vi "LowShooter Controller.vi"(8 "error in":errorcluster) -> ()   [LabVIEW 2015]
doc: "This VI executes continuously carrying out the current operation and responding to updates or new operations. It will often contain the timing or control code that is difficult to place directly in TeleOp. This VI generally opens all sensors and motors and isolates the rest of the robot code from knowing how the operations are carried out."
uses:
  LowShooter Operations.ctl
  <vilib>/Rock Robotics/WPI/CAN/TalonSRX/WPI_CANTalonSRX_GlobalStatus.ctl
  LowShooter Setpoints.ctl
  Framework/Motor Ref Names Type Def.ctl
  Solenoids/Solenoids.ctl
  <vilib>/Rock Robotics/WPI/Solenoid/WPI_SolenoidValue.ctl
  Framework/Robot Global Data.vi
  Shooter Global.vi
panel:
  out "Talon SRX Status":T1
  in  "OK Button":bool
  in  "Ball Seen":dbl
  out "Arm Down":bool
  out "Operation":T2
  out "Back Switch":bool
  out "Ball Present":bool
  out "error out":errorcluster
  in  "error in":errorcluster
  out "Current\nCmd 2":string
  out "Current\nCmd":string
  # "Tip: It may be helpful to observe inputs and sensor values.\nYou may also want to display tuning or debugging controls."
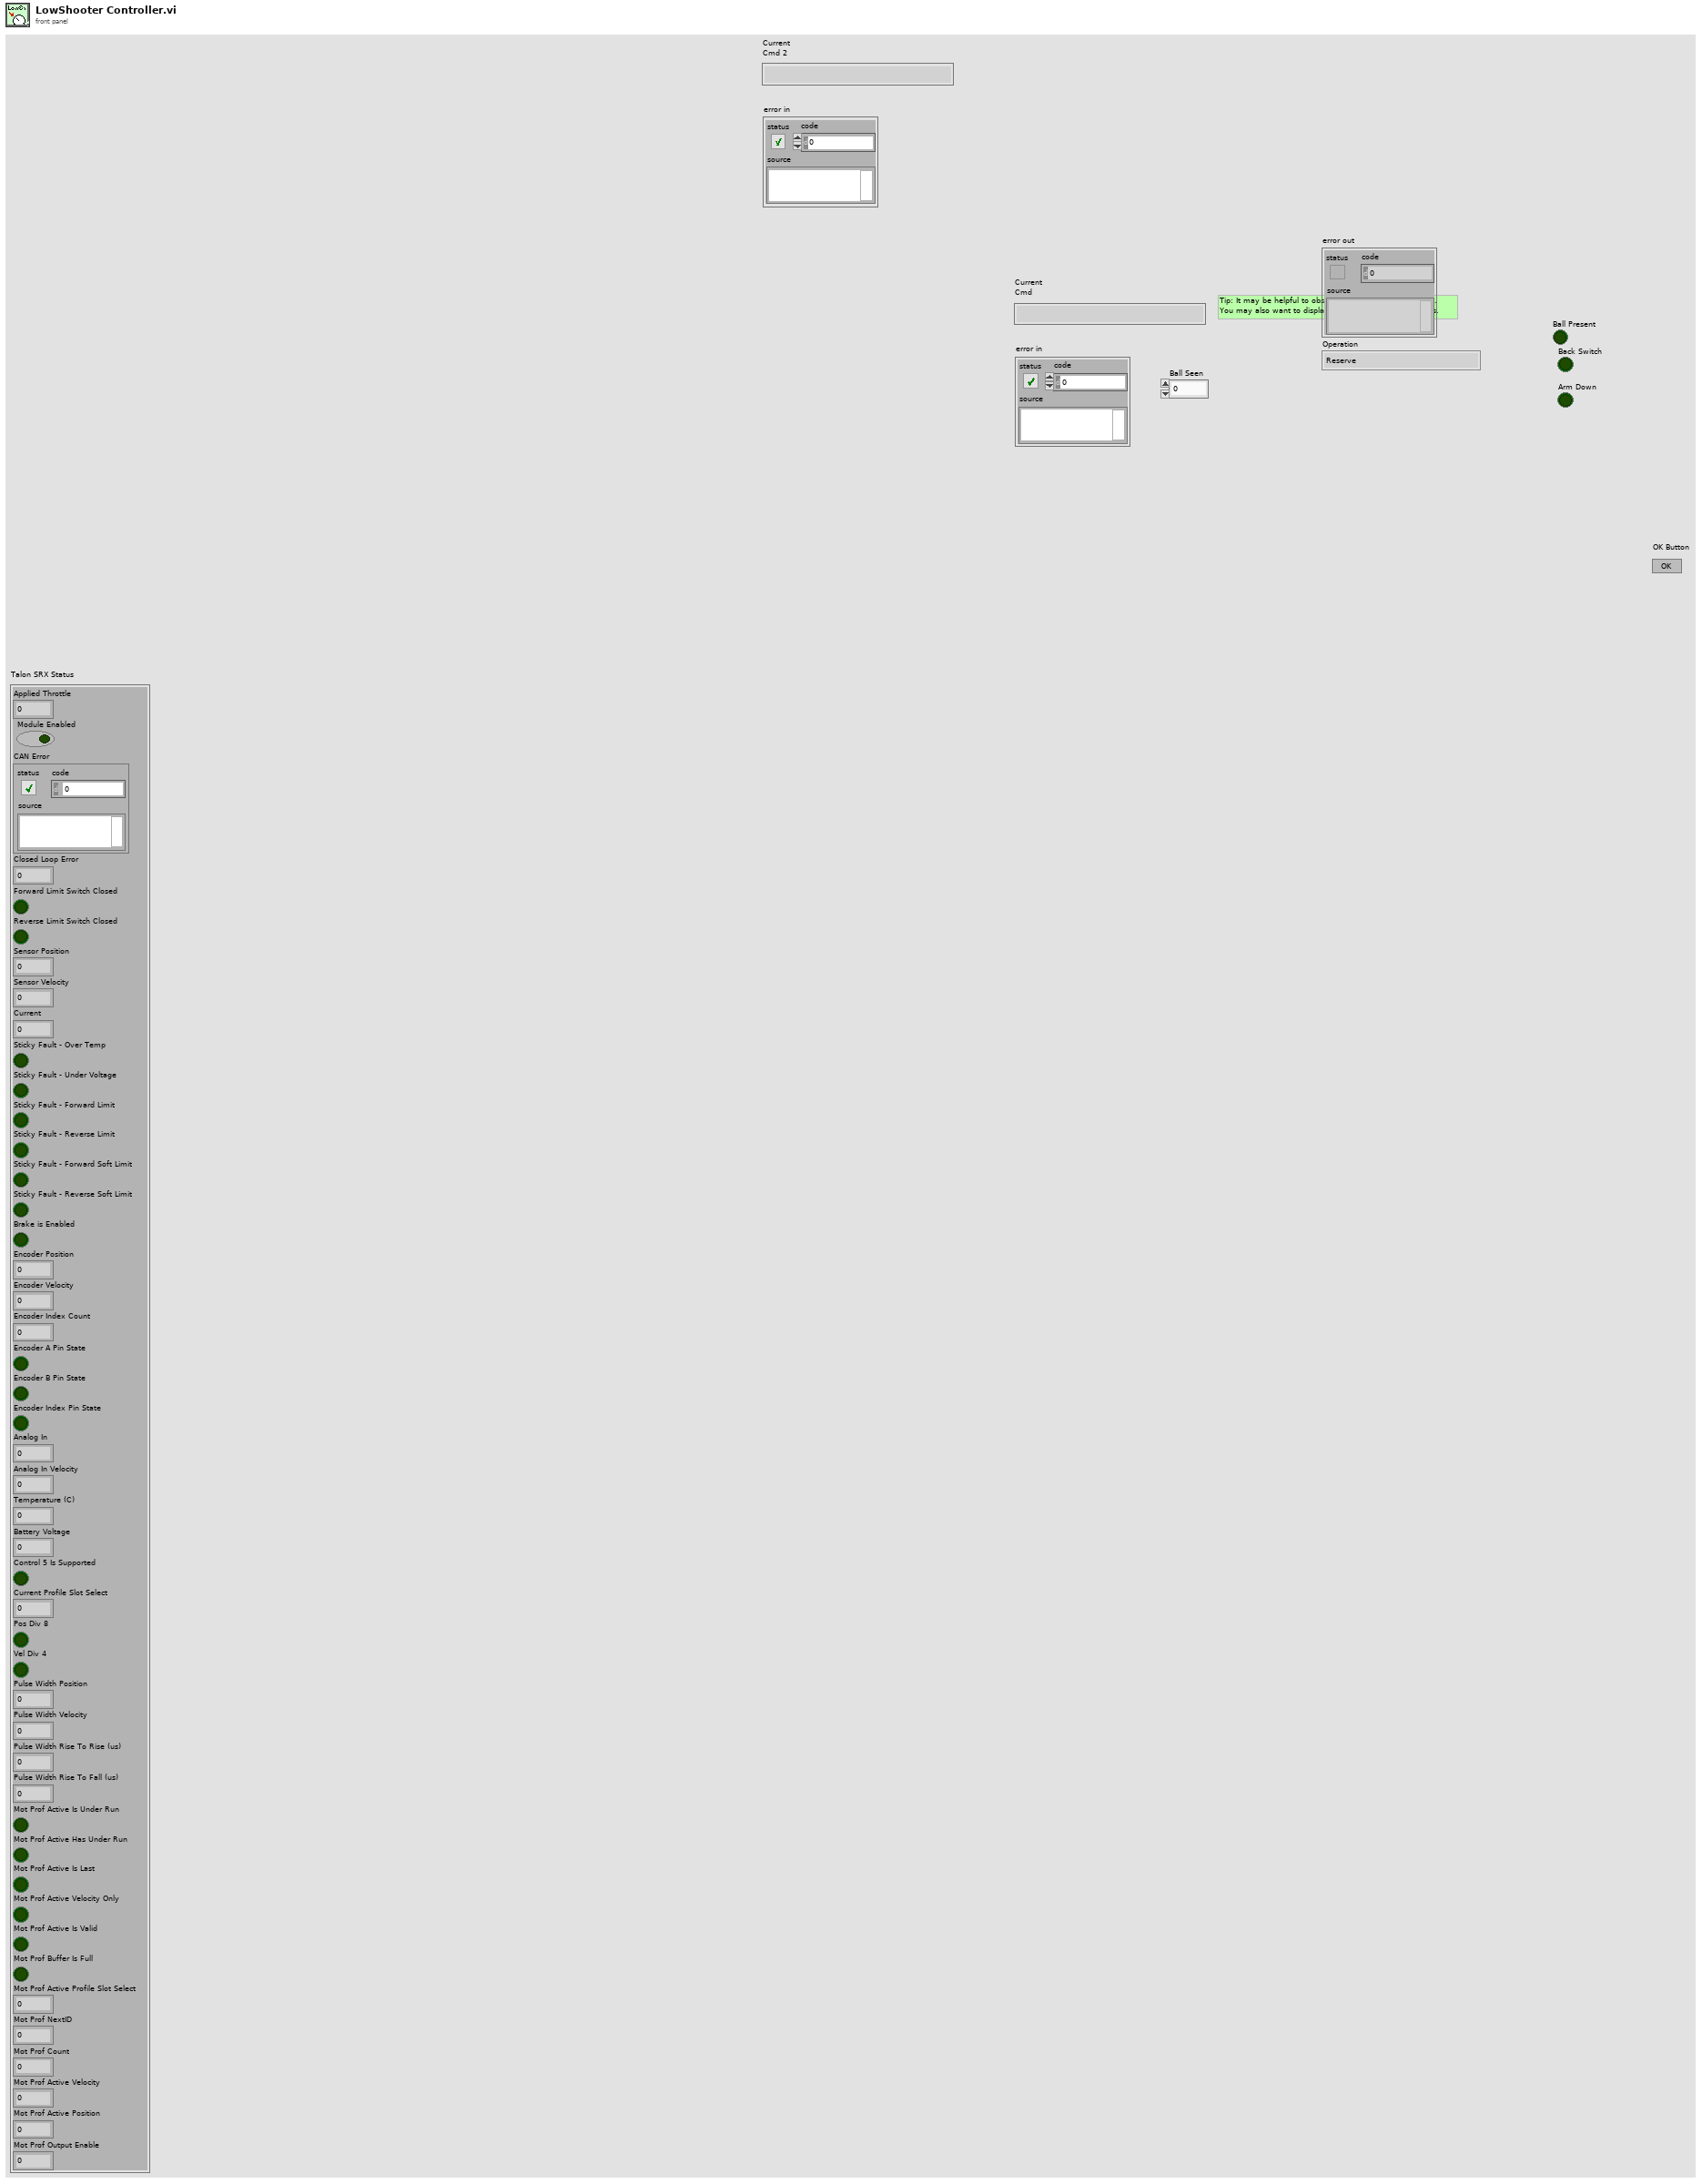
[diagram p1: front panel]
types:
  T1 = typedef "WPI_CANTalonSRX_GlobalStatus.ctl" = cluster{"Applied Throttle":dbl, "Module Enabled":bool, "CAN Error":errorcluster, "Closed Loop Error":dbl, "Forward Limit Switch Closed":bool, "Reverse Limit Switch Closed":bool, "Sensor Position":dbl, "Sensor Velocity":dbl, "Current":dbl, "Sticky Fault - Over Temp":bool, "Sticky Fault - Under Voltage":bool, "Sticky Fault - Forward Limit":bool, "Sticky Fault - Reverse Limit":bool, "Sticky Fault - Forward Soft Limit":bool, "Sticky Fault - Reverse Soft Limit":bool, "Brake is Enabled":bool, "Encoder Position":dbl, "Encoder Velocity":dbl, "Encoder Index Count":dbl, "Encoder A Pin State":bool, "Encoder B Pin State":bool, "Encoder Index Pin State":bool, "Analog In":dbl, "Analog In Velocity":dbl, "Temperature (C)":dbl, "Battery Voltage":dbl, "Control 5 Is Supported":bool, "Current Profile Slot Select":dbl, "Pos Div 8":bool, "Vel Div 4":bool, "Pulse Width Position":i32, "Pulse Width Velocity":i32, "Pulse Width Rise To Rise (us)":i32, "Pulse Width Rise To Fall (us)":i32, "Mot Prof Active Is Under Run":bool, "Mot Prof Active Has Under Run":bool, "Mot Prof Active Is Last":bool, "Mot Prof Active Velocity Only":bool, "Mot Prof Active Is Valid":bool, "Mot Prof Buffer Is Full":bool, "Mot Prof Active Profile Slot Select":i32, "Mot Prof NextID":i32, "Mot Prof Count":i32, "Mot Prof Active Velocity":dbl, "Mot Prof Active Position":dbl, "Mot Prof Output Enable":i32}
  T2 = typedef "LowShooter Operations.ctl" = enum16{"Reserve", "Read Current", "Immediate", "Shoot", "Retrieve", "Move Arm Down", "Move Arm"}
  T3 = typedef "Robot Type Def.ctl" = enum32{"Disabled", "Ghost", "Casper", "Lofty", "Board", "RaceRobot"}
  T4 = typedef "Motor Ref Names Type Def.ctl" = enum16{"Angular Motor", "Shooter Motor Bottom", "Shooter Motor Top", "Arm Shooter Motor"}
  T5 = typedef "WPI_SolenoidValue.ctl" = enum16{"Off", "On", "Forward", "Reverse"}
  T6 = typedef "Solenoids.ctl" = enum16{"Gear Low", "Gear High", "Shoot Ball", "Hold Ball", "PTO Active", "PTO De-Active"}
  T7 = typedef "LowShooter Setpoints.ctl" = cluster{"Operation":T2, "Setpoint":dbl, "Duration":dbl}
  T8 = typedef "Motor Ref Array Type Def.ctl" = T9[]
  T9 = typedef "Detailed Motor Type Def.ctl" = cluster{"MotorRef":T10, "Encoder Ticks Per Rev":dbl, "Set Position":dbl}
  T10 = typedef "WPI_MotorControlDeviceRef.ctl" = cluster{"DeviceStatus":errorcluster, "Type":T11, "PWM":cluster{"PWM Channel":T12, "DeadBand":T13}, "CAN":cluster{"Device Number":u8, "Control Mode":T14, "Semaphore":T15, "Max Vout":dbl, "TalonSRX Control Mode":T16}, "Invert":bool}
  T11 = typedef "WPI_MotorControlType.ctl" = enum16{"PWM", "CAN", "CANTalonSRX"}
  T12 = typedef "FPGA_DIOPWMChannel.ctl" = enum8{"PWM 0", "PWM 1", "PWM 2", "PWM 3", "PWM 4", "PWM 5", "PWM 6", "PWM 7", "PWM 8", "PWM 9", "PWM MXP 0", "PWM MXP 1", "PWM MXP 2", "PWM MXP 3", "PWM MXP 4", "PWM MXP 5", "PWM MXP 6", "PWM MXP 7", "PWM MXP 8", "PWM MXP 9", "Invalid"}
  T13 = typedef "WPI_PWMDeadband.ctl" = cluster{"Name":string, "maxPositivePwm":i32, "minPositivePwm":i32, "centerPwm":i32, "maxNegativePwm":i32, "minNegativePwm":i32, "angularRange":u16}
  T14 = typedef "WPI_CANJaguar_ControlMode.ctl" = enum8{"Percent VBus", "Current", "Speed", "Position", "Voltage"}
  T15 = typedef "Semaphore RefNum" = refnum<k1>
  T16 = typedef "WPI_CANTalonSRX_APIControlMode.ctl" = enum8{"Percent VBus", "Speed", "Position", "Slave", "Unchanged / Invalid", "Voltage Compensation", "Current", "Motion Profile"}
  T17 = typedef "Command Status Info.ctl" = cluster{"Name":string, "Status":T18, "notifier out":T19}
  T18 = typedef "Completion Status.ctl" = enum16{"Successful", "Aborted", "Incomplete"}
  T19 = typedef "Completion Notifier.ctl" = refnum<notifier>
  T20 = cluster{"Default Command":T7, "Command Timing":cluster{"Start Time (ms)":u32, "Iterations":i32}, "Command Arguments":cluster{"Command Info":T17, "Description":string, "Default Command":T7, "notifier out":refnum<notifier>, "Subsystem Name":string}}
  T21 = typedef "Addon Motor Type Def.ctl" = cluster{"SwitchDevRef":T22, "LidarRef":T25, "Arm Sensors":cluster{"Front Sensor":T22, "Back Sensor":T22, "Ball Sensor":T22}}
  T22 = typedef "WPI_SwitchDevRef.ctl" = cluster{"DevStatus":errorcluster, "DIO Channel":T23, "CntIndex":T24, "Normally Closed":bool}
  T23 = typedef "FPGA_DIOChannel.ctl" = enum8{"DIO 0", "DIO 1", "DIO 2", "DIO 3", "DIO 4", "DIO 5", "DIO 6", "DIO 7", "DIO 8", "DIO 9", "DIO MXP 0", "DIO MXP 1", "DIO MXP 2", "DIO MXP 3", "DIO MXP 4", "DIO MXP 5", "DIO MXP 6", "DIO MXP 7", "DIO MXP 8", "DIO MXP 9", "DIO MXP 10", "DIO MXP 11", "DIO MXP 12", "DIO MXP 13", "DIO MXP 14", "DIO MXP 15", "Invalid"}
  T24 = typedef "FPGA_CounterCtrSystemIndex.ctl" = enum8{"Ctr 0", "Ctr 1", "Ctr 2", "Ctr 3", "Ctr 4", "Ctr 5", "Ctr 6", "Ctr 7", "Invalid"}
  T25 = typedef "Lidar Type Def.ctl" = cluster{"I2CDevRef":T26}
  T26 = typedef "WPI_I2CDevRef.ctl" = cluster{"DevStatus":errorcluster, "Device Address":u8, "Handle":i32, "I2C Bus":T27}
  T27 = typedef "i2c_bus.ctl" = enum16{"I2C On-Board", "I2C MXP", "Invalid"}
  T28 = typedef "Shooter Settings Type Def.ctl" = cluster{"Bottom Roller Out Speed":dbl, "Top Roller Out Speed":dbl, "Bottom Roller In Speed":dbl, "Top Roller In Speed":dbl, "Intake Time Limit":dbl, "Intake Close Claw Delay":dbl, "Shoot Delay":dbl, "Shoot Follow Through":dbl}
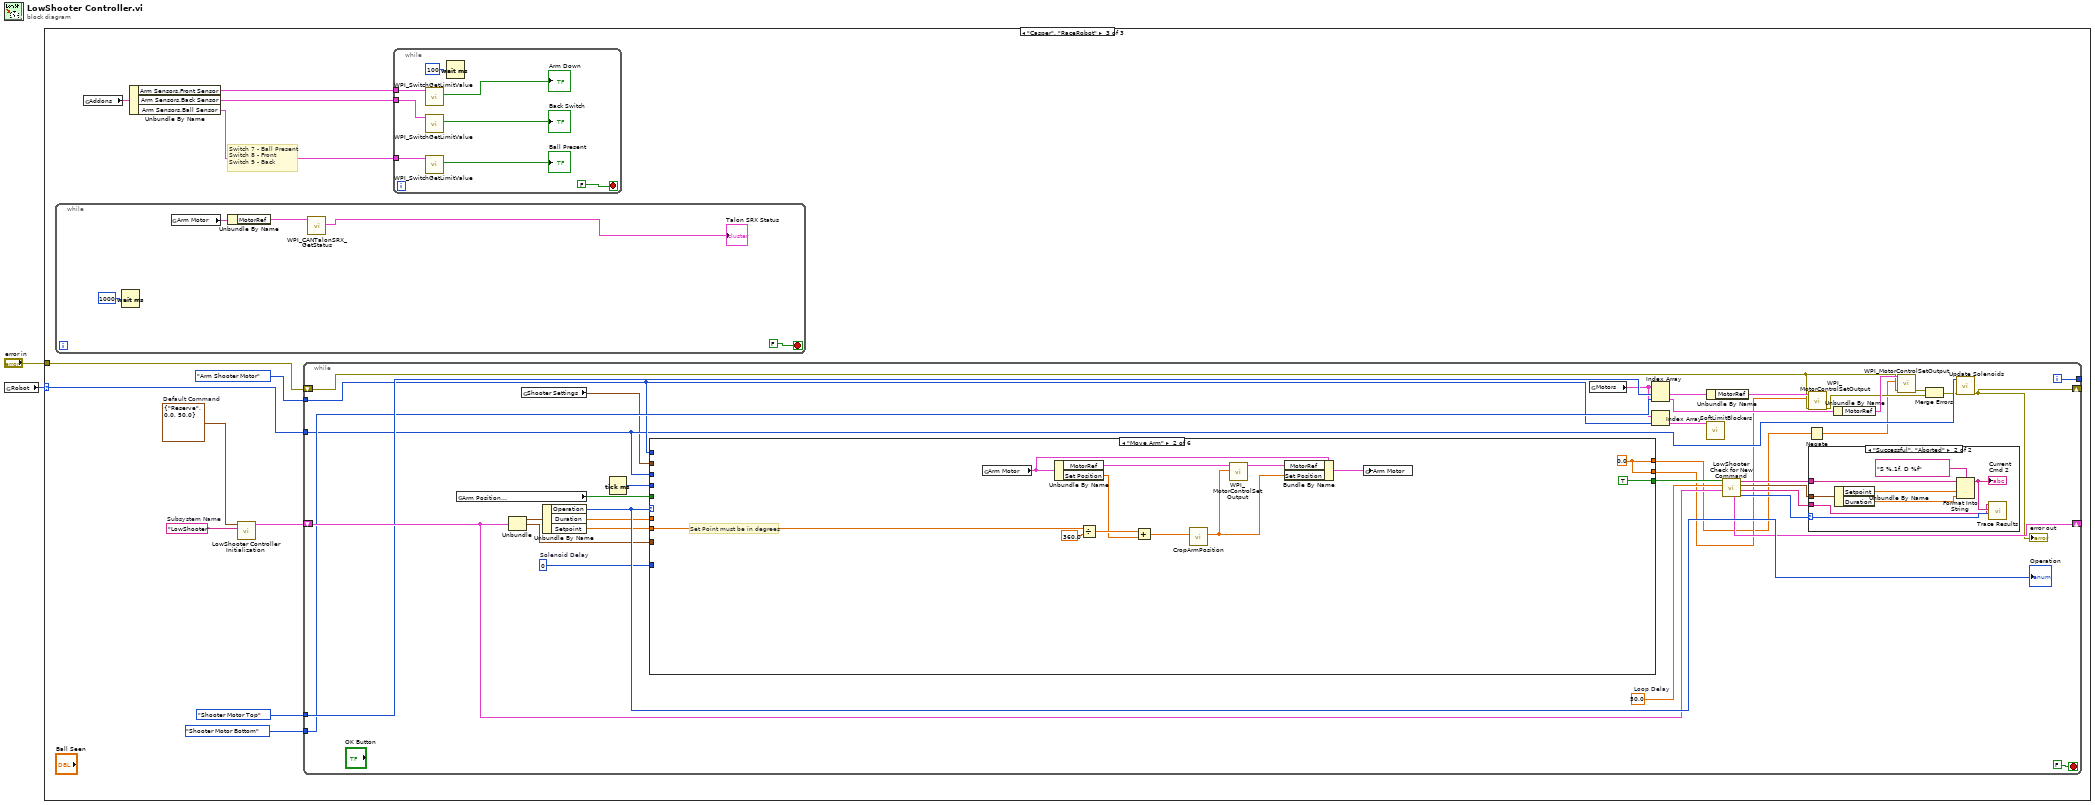
[diagram p0: block diagram]
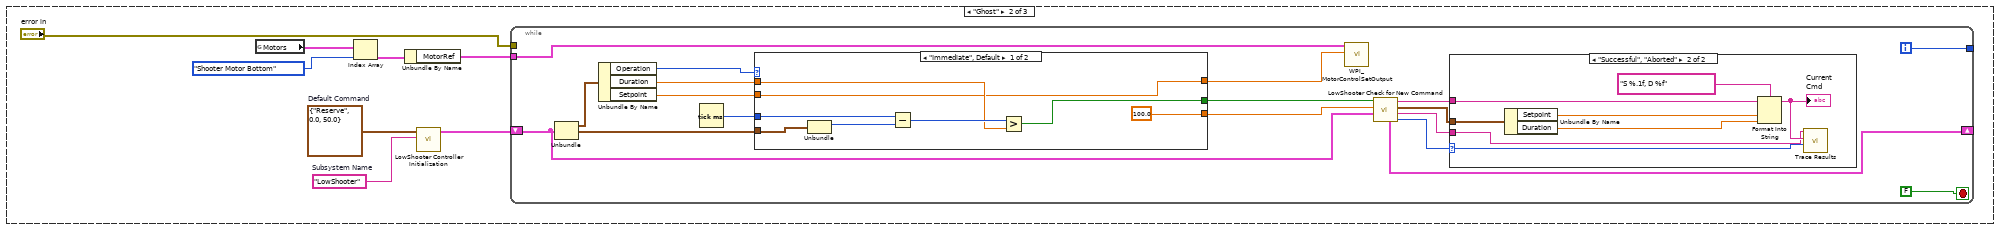
[diagram p3: hidden frame]
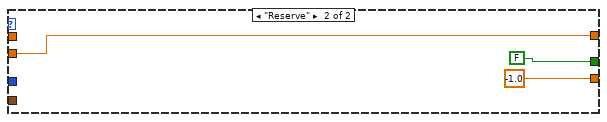
[diagram p5: hidden frame]
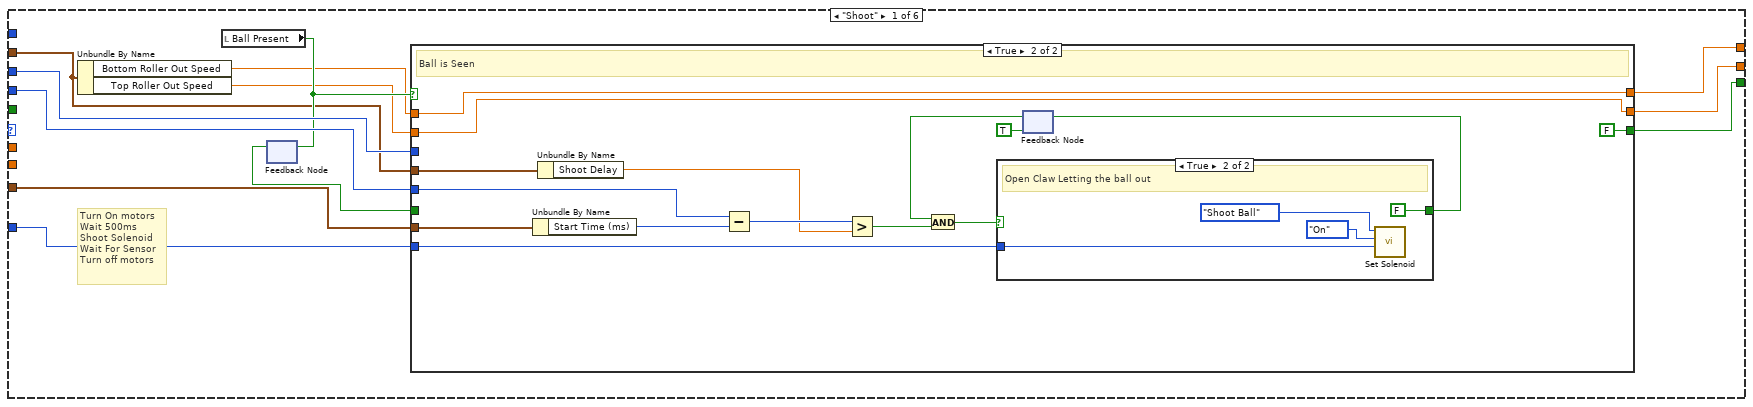
[diagram p7: hidden frame]
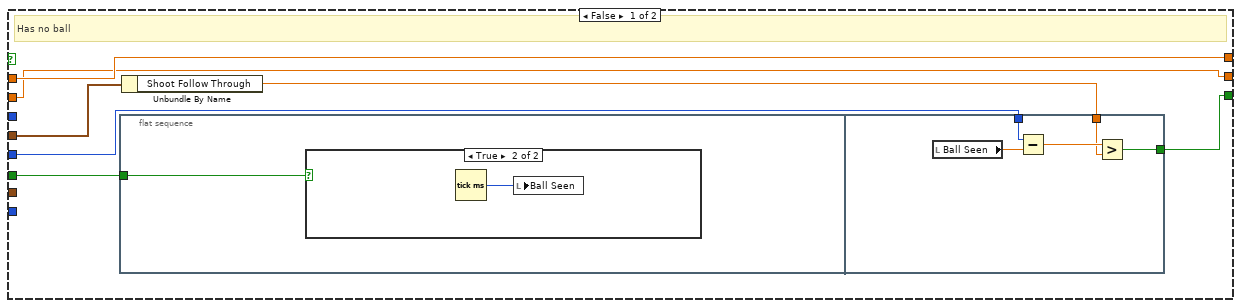
[diagram p8: hidden frame]
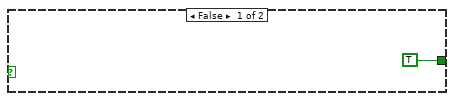
[diagram p10: hidden frame]
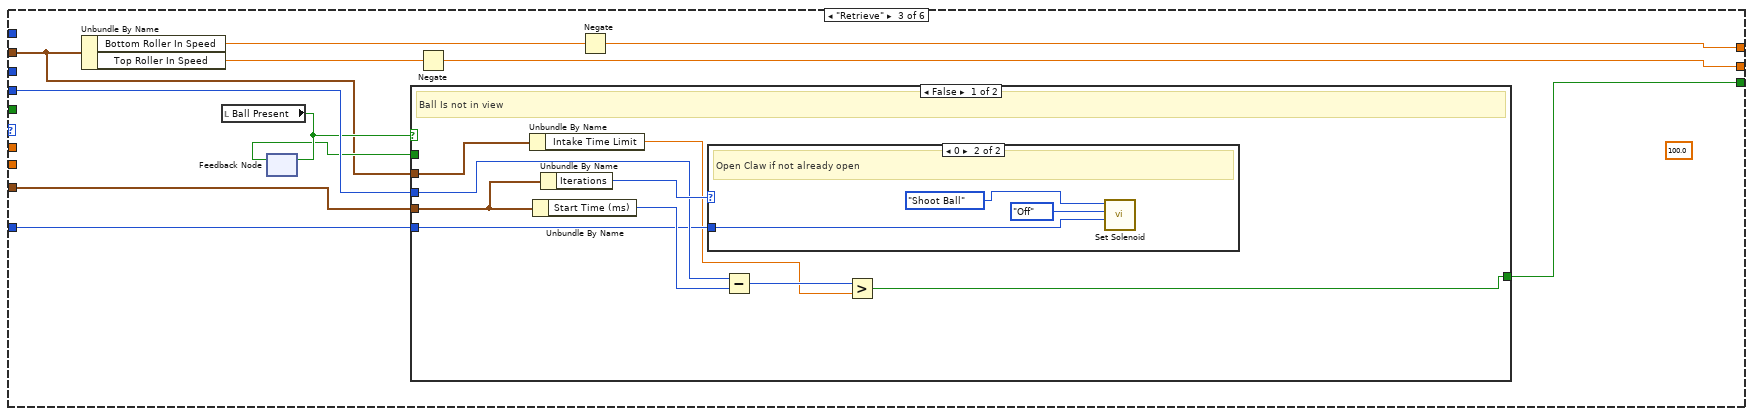
[diagram p11: hidden frame]
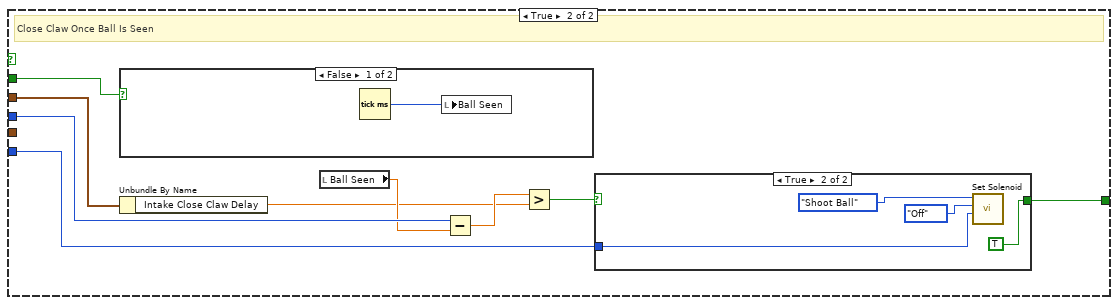
[diagram p13: hidden frame]
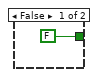
[diagram p14: hidden frame]
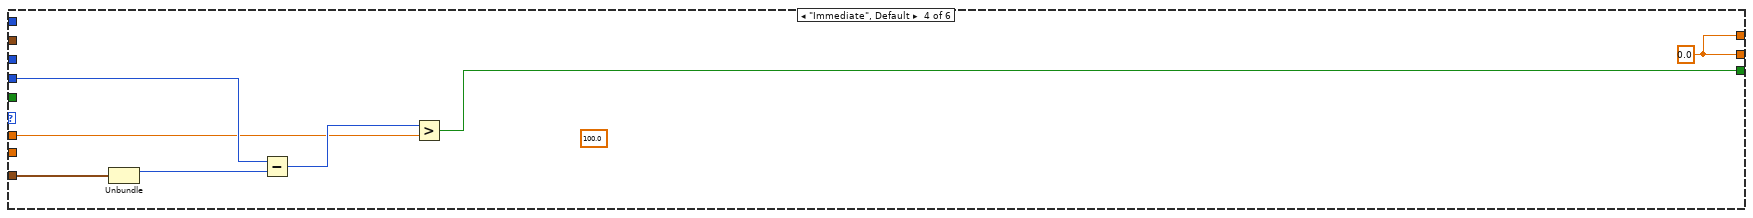
[diagram p16: hidden frame]
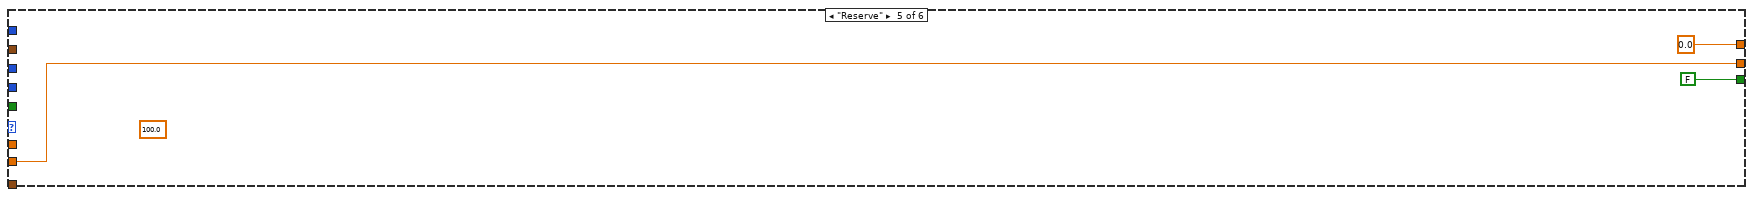
[diagram p17: hidden frame]
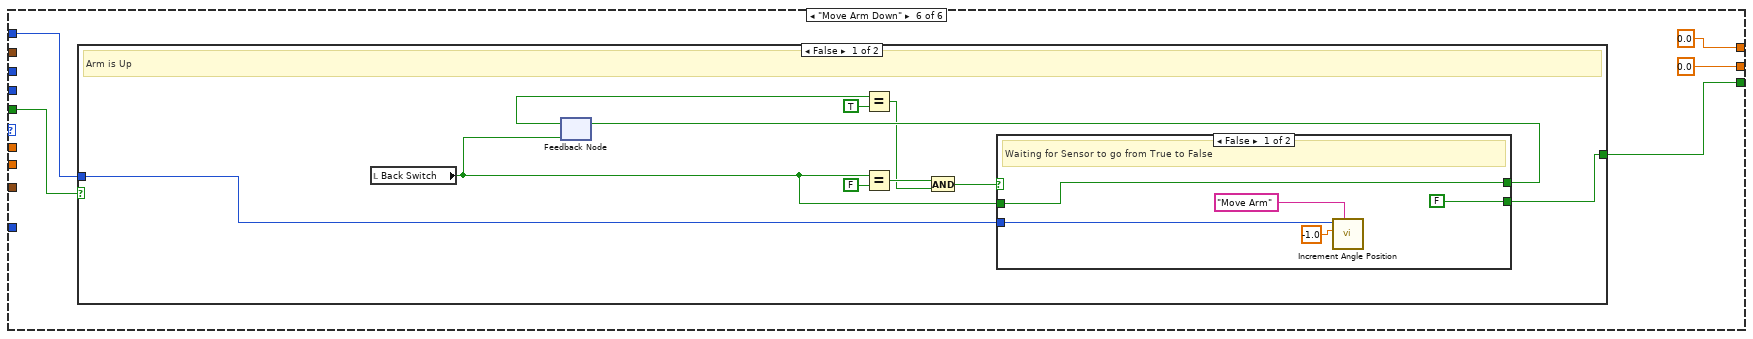
[diagram p18: hidden frame]
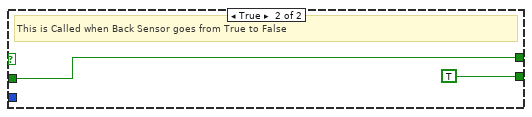
[diagram p19: hidden frame]
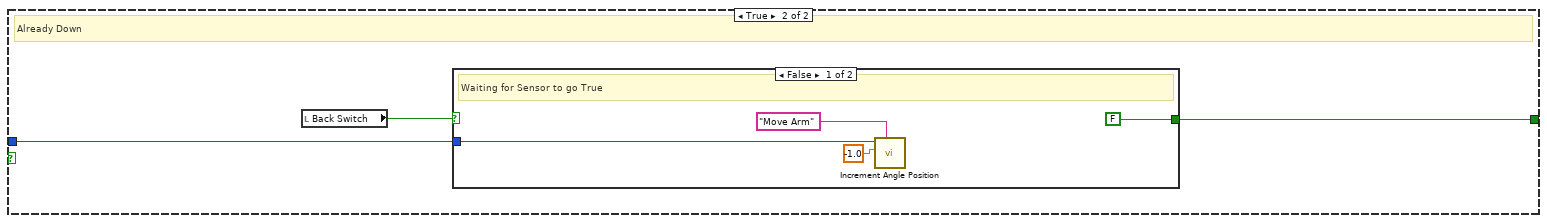
[diagram p20: hidden frame]
diagram:
  n1 = global read "Robot Global Data.vi" "Robot"() -> (w2:T3)
  n2 = case shown="\"Casper\", \"RaceRobot\"" w2 {
    selector: w2 -> [_ _ w48]
    tunnel: "error in" -> [_ _ w51]
    frame "Disabled", Default {
    }
    frame "Ghost" {
      w7 = T7 {"Operation"=enum."Reserve", "Setpoint"=0.0, "Duration"=50.0}  # Default Command
      w8 = "LowShooter"  # Subsystem Name
      n3 = global read "Robot Global Data.vi" "Motors"() -> (w6:T8)
      n4 = Index Array(array=w6, index=Motor_Ref_Names_Type_Def."Shooter Motor Bottom" ("Motor Ref Names")) -> (element=w5:T9)
      n5 = Unbundle By Name(w5) -> ("MotorRef"=w4:T10)
      n6 = call "LowShooter Controller Initialization.vi"("Subsystem Name"=w8, "Default Command"=w7) -> ("Command Info"=w9:T20)  [unwired: 9 in]
      n7 = while {
        shift-right: [w19] -> _
        shift-left: w9 -> [w20]
        tunnel: [w27] -> _
        tunnel: "error in" -> [_]
        tunnel: w4 -> [w11]
        i -> [w27]
        stop <- FALSE stop-if-true
        n8 = Unbundle(w20) -> ("Default Command"=w26:T7, "Command Timing"=w22:cluster{"Start Time (ms)":u32, "Iterations":i32})  [unwired: 1 out]
        n9 = Unbundle By Name(w26) -> ("Operation"=w25:T2, "Duration"=w24:dbl, "Setpoint"=w21:dbl)
        n10 = Tick Count (ms)() -> (millisecond timer value=w23:u32)
        n11 = case shown="\"Immediate\", Default" w25 {
          tunnel: [100.0 -1.0] -> w17
          tunnel: [w39 FALSE ("ignore previous (F)")] -> w18
          tunnel: w22 -> [w41 _]
          tunnel: w24 -> [w38 _]
          tunnel: w23 -> [w40 _]
          tunnel: w21 -> [w37 w45]
          tunnel: [w37 w45] -> w12
          frame "Immediate", Default {
            n12 = Unbundle(w41) -> ("Start Time (ms)"=w43:u32)  [unwired: 1 out]
            n13 = Subtract(x=w40, y=w43) -> (x-y=w42:u32)
            n14 = Greater?(x=w42, y=w38) -> (0:w39:bool)
          }
          frame "Reserve" {
          }
        }
        n15 = call <vilib>:"WPI_MotorControlSetOutput.vi"("Output"=w12, "MotorControlDevRef"=w11) -> ()  [unwired: 7 in, 3 out]
        n16 = call "LowShooter Check for New Command.vi"("Current Command"=w20, "Wait time (ms)"=w17, "Finished?"=w18) -> ("Completion"=w13:T18, "Subsystem Name"=w14:string, "Current Command"=w15:T7, "Initial Trace String"=w16:string, "NextCommand"=w19:T20)  [unwired: 4 in]
        n17 = case shown="\"Successful\", \"Aborted\"" w13 {
          selector: w13 -> [_ w36]
          tunnel: w16 -> [_ w32]
          tunnel: w15 -> [_ w33]
          tunnel: w14 -> [_ w29]
          frame "Incomplete", Default {
            # "Continuing current command"
          }
          frame "Successful", "Aborted" {
            # "Report and setup for next command"
            n18 = Unbundle By Name(w33) -> ("Setpoint"=w35:dbl, "Duration"=w30:dbl)
            n19 = Format Into String(format string="S %.1f, D %f", initial string=w32, w35, w30) -> (resulting string=w31:string)  [unwired: 1 in, 1 out]
            "Current\nCmd" <- w31
            n20 = call <vilib>:"Trace Results.vi"("Status of previous command"=w36, "Description"=w31, "Subsystem"=w29) -> ()  [unwired: 9 in]
          }
        }
      }
    }
    frame "Casper", "RaceRobot" {
      w58 = T7 {"Operation"=enum."Reserve", "Setpoint"=0.0, "Duration"=50.0}  # Default Command
      w57 = "LowShooter"  # Subsystem Name
      # "Switch 7 - Ball Present\nSwitch 8 - Front\nSwitch 9 - Back"
      n21 = while {
        stop <- FALSE stop-if-true
        n22 = Wait (ms)(milliseconds to wait=u32 1000) -> ()  [unwired: 1 out]
        n23 = global read "Shooter Global.vi" "Arm Motor"() -> (w64:T9)
        n24 = Unbundle By Name(w64) -> ("MotorRef"=w63:T10)
        n25 = call <vilib>:"WPI_CANTalonSRX_GetStatus.vi"("CAN Talon SRX Ref"=w63) -> ("Talon SRX Status"=→"Talon SRX Status":T1)  [unwired: 8 in, 2 out]
      }
      n26 = global read "Robot Global Data.vi" "Addons"() -> (w54:T21)
      n27 = Unbundle By Name(w54) -> ("Arm Sensors.Front Sensor"=w49:T22, "Arm Sensors.Back Sensor"=w52:T22, "Arm Sensors.Ball Sensor"=w53:T22)
      n28 = call "LowShooter Controller Initialization.vi"("Subsystem Name"=w57, "Default Command"=w58) -> ("Command Info"=w56:T20)  [unwired: 9 in]
      n29 = while {
        shift-right: [w100] -> _
        shift-left: w56 -> [w101]
        tunnel: [w108] -> _
        tunnel: Motor_Ref_Names_Type_Def."Shooter Motor Top" ("Motor Ref Names") -> [w92]
        shift-right: [w86] -> _
        shift-left: w51 -> [w78]
        tunnel: Motor_Ref_Names_Type_Def."Arm Shooter Motor" ("Motor Ref Names") -> [w84]
        tunnel: Motor_Ref_Names_Type_Def."Shooter Motor Bottom" ("Motor Ref Names") -> [w88]
        tunnel: w48 -> [w82]
        i -> [w108]
        stop <- FALSE stop-if-true
        w83 = 50.0  # Loop Delay
        w87 = 0  # Solenoid Delay
        n30 = global read "Robot Global Data.vi" "Arm Position \nUp = Down\nDown = Up"() -> (w91:bool)
        n31 = Unbundle(w101) -> ("Default Command"=w107:T7, "Command Timing"=w103:cluster{"Start Time (ms)":u32, "Iterations":i32})  [unwired: 1 out]
        n32 = global read "Shooter Global.vi" "Shooter Settings"() -> (w77:T28)
        n33 = Unbundle By Name(w107) -> ("Operation"=w106:T2, "Duration"=w105:dbl, "Setpoint"=w102:dbl)
        "Operation" <- w106
        n34 = Tick Count (ms)() -> (millisecond timer value=w104:u32)
        n35 = case shown="\"Move Arm\"" w106 {
          tunnel: [w129 TRUE ("ignore previous (F)") w185 w216 FALSE ("ignore previous (F)") w225] -> w99
          tunnel: w103 -> [w128 _ w186 w218 _ _]
          tunnel: w105 -> [_ _ _ w215 _ _]
          tunnel: w104 -> [w127 _ w184 w217 _ _]
          tunnel: w102 -> [_ w172 _ _ w222 _]
          tunnel: [w124 w175 w179 w214 w222 0.0 ("Setpoint")] -> w75
          tunnel: w84 -> [_ _ _ _ _ w228]
          tunnel: w91 -> [_ _ _ _ _ w226]
          tunnel: [w125 w175 w180 w214 0.0 ("Numeric") 0.0 ("Numeric")] -> w73
          tunnel: w87 -> [w126 _ w181 _ _ _]
          tunnel: w82 -> [w123 _ _ _ _ _]
          tunnel: w77 -> [w118 _ w176 _ _ _]
          frame "Shoot" {
            # "Turn On motors\nWait 500ms\nShoot Solenoid\nWait For Sensor\nTurn off motors"
            n36 = Unbundle By Name(w118) -> ("Bottom Roller Out Speed"=w119:dbl, "Top Roller Out Speed"=w120:dbl)
            n37 = local read "Ball Present"() -> (w122:bool)
            n38 = feedback #1() -> (w121:bool)  [unwired: 1 in]
            n39 = feedback-in #1(w122) -> ()
            n40 = case shown="True" w122 {
              tunnel: [w135 FALSE ("ignore previous (F)")] -> w129
              tunnel: w128 -> [_ w158]
              tunnel: w127 -> [w134 w156]
              tunnel: w126 -> [_ w148]
              tunnel: w119 -> [w133 w147]
              tunnel: [w133 w147] -> w125
              tunnel: w120 -> [w132 w146]
              tunnel: [w132 w146] -> w124
              tunnel: w123 -> [_ _]
              tunnel: w121 -> [w136 _]
              tunnel: w118 -> [w131 w144]
              frame False {
                # "Has no ball"
                n41 = flat-sequence {
                  tunnel: w136 -> [w137]
                  tunnel: [w141] -> w135
                  tunnel: w134 -> [w140]
                  tunnel: w130 -> [w139]
                  frame #0 {
                    n42 = case shown="True" w137 {
                      frame False {
                      }
                      frame True {
                        n43 = Tick Count (ms)() -> (millisecond timer value=w138:u32)
                        n44 = local write "Ball Seen"(w138) -> ()
                      }
                    }
                  }
                  frame #1 {
                    n45 = local read "Ball Seen"() -> (w143:dbl)
                    n46 = Subtract(x=w140, y=w143) -> (x-y=w142:dbl)
                    n47 = Greater?(x=w142, y=w139) -> (0:w141:bool)
                  }
                }
                n48 = Unbundle By Name(w131) -> ("Shoot Follow Through"=w130:dbl)
              }
              frame True {
                # "Ball is Seen"
                n49 = Unbundle By Name(w158) -> ("Start Time (ms)"=w157:u32)
                n50 = Unbundle By Name(w144) -> ("Shoot Delay"=w145:dbl)
                n51 = Subtract(x=w156, y=w157) -> (x-y=w155:u32)
                n52 = Greater?(x=w155, y=w145) -> (0:w153:bool)
                n53 = feedback #2(TRUE) -> (w151:bool)
                n54 = And(x=w151, y=w153) -> (x .and. y?=w154:bool)
                n55 = case shown="True" w154 {
                  tunnel: [TRUE FALSE] -> w152
                  tunnel: w148 -> [_ w162]
                  frame False {
                  }
                  frame True {
                    # "Open Claw Letting the ball out"
                    n56 = call "Set Solenoid.vi"("On For (0 = Forever)"=w162, "Value"=WPI_SolenoidValue."On", "Solenoids"=Solenoids."Shoot Ball") -> ()  [unwired: 8 in, 1 out]
                  }
                }
                n57 = feedback-in #2(w152) -> ()
              }
            }
          }
          frame "Move Arm" {
            w175 = 0.0
            # "Set Point must be in degrees"
            n58 = global read "Shooter Global.vi" "Arm Motor"() -> (w173:T9)
            n59 = Unbundle By Name(w173) -> ("MotorRef"=w168:T10, "Set Position"=w169:dbl)
            n60 = Divide(x=w172, y=360.0) -> (x/y=w170:dbl)
            n61 = Add(x=w170, y=w169) -> (x+y=w164:dbl)
            n62 = call "CropArmPosition.vi"("Position"=w164) -> ("New Position"=w165:dbl)  [unwired: 10 in]
            n63 = call <vilib>:"WPI_MotorControlSetOutput.vi"("Output"=w165, "MotorControlDevRef"=w168) -> ("MotorControlDevRef"=w167:T10)  [unwired: 7 in, 2 out]
            n64 = Bundle By Name(cluster=w173, "MotorRef"=w167, "Set Position"=w165) -> (w166:T9)
            n65 = global write "Shooter Global.vi" "Arm Motor"(w166) -> ()
          }
          frame "Retrieve" {
            (unwired) 100.0
            n66 = Unbundle By Name(w176) -> ("Bottom Roller In Speed"=w178:dbl, "Top Roller In Speed"=w177:dbl)
            n67 = local read "Ball Present"() -> (w183:bool)
            n68 = feedback-in #3(w183) -> ()
            n69 = feedback #3() -> (w182:bool)  [unwired: 1 in]
            n70 = case shown="False" w183 {
              tunnel: w186 -> [w190 _]
              tunnel: [w192 w202] -> w185
              tunnel: w184 -> [w191 w204]
              tunnel: w182 -> [_ w207]
              tunnel: w181 -> [w189 w201]
              tunnel: w176 -> [w188 w200]
              frame False {
                # "Ball Is not in view"
                n71 = Unbundle By Name(w188) -> ("Intake Time Limit"=w187:dbl)
                n72 = Unbundle By Name(w190) -> ("Start Time (ms)"=w194:u32)
                n73 = Unbundle By Name(w190) -> ("Iterations"=w195:i32)
                n74 = case shown="0" w195 {
                  tunnel: w189 -> [_ w198]
                  frame Default {
                  }
                  frame 0 {
                    # "Open Claw if not already open"
                    n75 = call "Set Solenoid.vi"("On For (0 = Forever)"=w198, "Value"=WPI_SolenoidValue."Off", "Solenoids"=Solenoids."Shoot Ball") -> ()  [unwired: 8 in, 1 out]
                  }
                }
                n76 = Subtract(x=w191, y=w194) -> (x-y=w193:u32)
                n77 = Greater?(x=w193, y=w187) -> (0:w192:bool)
              }
              frame True {
                # "Close Claw Once Ball Is Seen"
                n78 = case shown="False" w207 {
                  frame False {
                    n79 = Tick Count (ms)() -> (millisecond timer value=w213:u32)
                    n80 = local write "Ball Seen"(w213) -> ()
                  }
                  frame True {
                  }
                }
                n81 = Unbundle By Name(w200) -> ("Intake Close Claw Delay"=w199:dbl)
                n82 = local read "Ball Seen"() -> (w203:dbl)
                n83 = Subtract(x=w204, y=w203) -> (x-y=w206:dbl)
                n84 = Greater?(x=w206, y=w199) -> (0:w205:bool)
                n85 = case shown="True" w205 {
                  tunnel: [FALSE ("ignore previous (F)") TRUE ("ignore previous (F)")] -> w202
                  tunnel: w201 -> [_ w212]
                  frame False {
                  }
                  frame True {
                    n86 = call "Set Solenoid.vi"("On For (0 = Forever)"=w212, "Value"=WPI_SolenoidValue."Off", "Solenoids"=Solenoids."Shoot Ball") -> ()  [unwired: 8 in, 1 out]
                  }
                }
              }
            }
            n87 = Negate(x=w177) -> (-x=w179:dbl)
            n88 = Negate(x=w178) -> (-x=w180:dbl)
          }
          frame "Immediate", Default {
            w214 = 0.0
            (unwired) 100.0
            n89 = Unbundle(w218) -> ("Start Time (ms)"=w220:u32)  [unwired: 1 out]
            n90 = Subtract(x=w217, y=w220) -> (x-y=w219:u32)
            n91 = Greater?(x=w219, y=w215) -> (0:w216:bool)
          }
          frame "Reserve" {
            (unwired) 100.0
          }
          frame "Move Arm Down" {
            n92 = case shown="False" w226 {
              tunnel: w228 -> [w238 w248]
              tunnel: [w237 w247] -> w225
              frame False {
                # "Arm is Up"
                n93 = local read "Back Switch"() -> (w232:bool)
                n94 = feedback #4(w232) -> (w229:bool)
                n95 = Equal?(x=w229, y=TRUE) -> (x = y?=w231:bool)
                n96 = Equal?(x=w232, y=FALSE) -> (x = y?=w235:bool)
                n97 = And(x=w235, y=w231) -> (x .and. y?=w234:bool)
                n98 = case shown="False" w234 {
                  tunnel: w238 -> [w241 _]
                  tunnel: [FALSE TRUE] -> w237
                  tunnel: [w239 w244] -> w233
                  tunnel: w232 -> [w239 w244]
                  frame False {
                    # "Waiting for Sensor to go from True to False"
                    n99 = call "Increment Angle Position.vi"("Description"="Move Arm", "Angle"=-1.0, "Motor ID"=w241) -> ()  [unwired: 8 in, 1 out]
                  }
                  frame True {
                    # "This is Called when Back Sensor goes from True to False"
                  }
                }
                n100 = feedback-in #4(w233) -> ()
              }
              frame True {
                # "Already Down"
                n101 = local read "Back Switch"() -> (w246:bool)
                n102 = case shown="False" w246 {
                  tunnel: [FALSE TRUE] -> w247
                  tunnel: w248 -> [w249 _]
                  frame False {
                    # "Waiting for Sensor to go True"
                    n103 = call "Increment Angle Position.vi"("Description"="Move Arm", "Angle"=-1.0, "Motor ID"=w249) -> ()  [unwired: 8 in, 1 out]
                  }
                  frame True {
                    # "Waits for the sensor to be True"
                  }
                }
              }
            }
          }
        }
        n104 = global read "Robot Global Data.vi" "Motors"() -> (w85:T8)
        n105 = Index Array(array=w85, index #1=w92, index #2=w88) -> (element #1=w93:T9, element #2=w89:T9)
        n106 = Index Array(array=w85, index=w84) -> (element=w76:T9)
        n107 = Unbundle By Name(w93) -> ("MotorRef"=w94:T10)
        n108 = call "SoftLimitBlockers.vi"("Motor Ref"=w76) -> ()  [unwired: 11 in]
        n109 = call "LowShooter Check for New Command.vi"("Current Command"=w101, "Wait time (ms)"=w83, "Finished?"=w99) -> ("Completion"=w95:T18, "Subsystem Name"=w96:string, "Current Command"=w97:T7, "Initial Trace String"=w98:string, "NextCommand"=w100:T20)  [unwired: 4 in]
        n110 = Negate(x=w73) -> (-x=w74:dbl)
        n111 = call <vilib>:"WPI_MotorControlSetOutput.vi"("error in (no error)"=w78, "Output"=w75, "MotorControlDevRef"=w94) -> ("error out"=w79:errorcluster)  [unwired: 6 in, 2 out]
        n112 = case shown="\"Successful\", \"Aborted\"" w95 {
          selector: w95 -> [_ w117]
          tunnel: w98 -> [_ w113]
          tunnel: w97 -> [_ w114]
          tunnel: w96 -> [_ w110]
          frame "Incomplete", Default {
            # "Continuing current command"
          }
          frame "Successful", "Aborted" {
            # "Report and setup for next command"
            n113 = Unbundle By Name(w114) -> ("Setpoint"=w116:dbl, "Duration"=w111:dbl)
            n114 = Format Into String(format string="S %.1f, D %f", initial string=w113, w116, w111) -> (resulting string=w112:string)  [unwired: 1 in, 1 out]
            "Current\nCmd 2" <- w112
            n115 = call <vilib>:"Trace Results.vi"("Status of previous command"=w117, "Description"=w112, "Subsystem"=w110) -> ()  [unwired: 9 in]
          }
        }
        n116 = Unbundle By Name(w89) -> ("MotorRef"=w90:T10)
        n117 = call <vilib>:"WPI_MotorControlSetOutput.vi"("error in (no error)"=w78, "Output"=w74, "MotorControlDevRef"=w90) -> ("error out"=w81:errorcluster)  [unwired: 6 in, 2 out]
        n118 = Merge Errors(w81, w79) -> (w80:errorcluster)
        n119 = call "Update Solenoids.vi"("error in (no error)"=w80, "Robot"=w82) -> ("error out"=w86:errorcluster)  [unwired: 9 in]
        "error out" <- w86
      }
      n120 = while {
        tunnel: w53 -> [w68]
        tunnel: w52 -> [w67]
        tunnel: w49 -> [w66]
        stop <- FALSE stop-if-true
        n121 = call <vilib>:"WPI_SwitchGetLimitValue.vi"("SwitchDevRef"=w66) -> ("Switch Pressed"=→"Arm Down":bool)  [unwired: 8 in, 2 out]
        n122 = call <vilib>:"WPI_SwitchGetLimitValue.vi"("SwitchDevRef"=w67) -> ("Switch Pressed"=→"Back Switch":bool)  [unwired: 8 in, 2 out]
        n123 = call <vilib>:"WPI_SwitchGetLimitValue.vi"("SwitchDevRef"=w68) -> ("Switch Pressed"=→"Ball Present":bool)  [unwired: 8 in, 2 out]
        n124 = Wait (ms)(milliseconds to wait=u32 100) -> ()  [unwired: 1 out]
      }
    }
  }
